vi "configureWaveformType.vi"(0 "NInstrSim":refnum<class "NInstrSim.lvclass">, 2 "function (0:Sine)":u16(ring) items=["Sine", "Square", "Sine+Noise", "Random", "Chirp"], 5 "error in (no error)":errorcluster) -> (14 "dup NInstrSim":refnum<class "NInstrSim.lvclass">, 19 "error out":errorcluster)   [LabVIEW 2009, in "HB_Device_Examples.lvlib" / "NInstrSim.lvclass"]
doc: "Configures the waveform type generated by the NI Instrument Simulator."
uses:
  NInstrSim.lvclass
  non_GPL/instr.lib/NI Instrument Simulator/NI Instrument Simulator.lvlib
  lib.lib/HGF_LVC/HGF_DeviceBaseClasses/HGF_VISADevice/HGF_VISADevice.lvclass
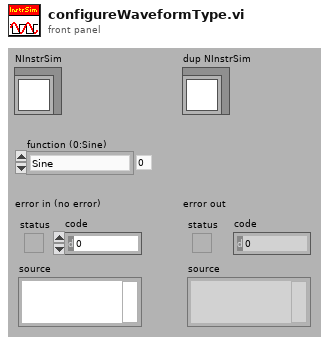
[diagram p1: front panel]
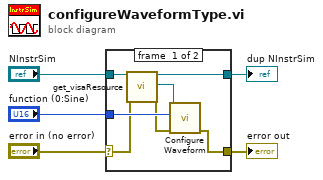
[diagram p0: block diagram]
diagram:
  n1 = case shown="No Error" "error in (no error)" {
    selector: "error in (no error)" -> [w7 w14]
    tunnel: [w6 w14] -> w4
    tunnel: [w11 w13] -> w2
    tunnel: "NInstrSim" -> [w12 w13]
    tunnel: "function (0:Sine)" -> [w9 _]
    frame #0 {
      n2 = call "get_visaResource.vi"("HGF_VISADevice"=w12, "error in (no error)"=w7) -> ("dup HGF_VISADevice"=w11:refnum<class "NInstrSim.lvclass">, "VISA Resource Name"=w10:refnum<visa-resource-name>, "error out"=w8:errorcluster)  [unwired: 15 out]
      n3 = call "Configure Waveform.vi"("error in (no error)"=w8, "Waveform Function (0:Sine)"=w9, "VISA resource name"=w10) -> ("error out"=w6:errorcluster)  [unwired: 8 out]
    }
    frame #1 {
    }
  }
  "error out" <- w4
  "dup NInstrSim" <- w2
